vi "noise_floor.vi"(9 "Last bin":i32, 10 "First bin":i32, 11 "FFT":cdb[](array[numeric])) -> (3 "Noise floor":dbl)   [LabVIEW 2014]
panel:
  # "We'll take the noise floor of a spectrum to be the median of the bins.  This is useful both to find the true noise floor and to see if a spectrum has been corrupted by impulse noise or large low frequency content."
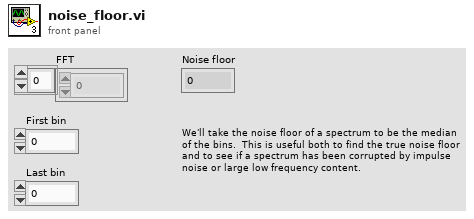
[diagram p1: front panel]
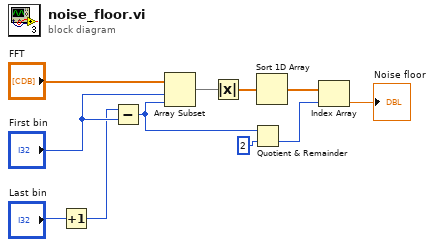
[diagram p0: block diagram]
diagram:
  n1 = Increment(x="Last bin") -> (x+1=w4:i32)
  n2 = Subtract(x=w4, y="First bin") -> (x-y=w7:i32)
  n3 = Array Subset(array="FFT", index="First bin", length=w7) -> (w9:cdb[])
  n4 = Absolute Value(x=w9) -> (abs(x)=w8:dbl[])
  n5 = Quotient & Remainder(x=w7, y=2) -> (floor(x/y)=w2:i32)  [unwired: 1 out]
  n6 = Sort 1D Array(array=w8) -> (sorted array=w3:dbl[])
  n7 = Index Array(array=w3, index=w2) -> (element=→"Noise floor":dbl)
